vi "Get ObjFlags.vi"(11 "Object Type in":refnum<class "Object Type Base.lvclass">) -> (1 "Set?":bool, 2 "ObjFlags":u32, 3 "Object Type out":refnum<class "Object Type Base.lvclass">)   [LabVIEW 2024, in "EDS.lvlib" / "Object Type Base.lvclass"]
uses:
  Object Type Base.lvclass
  Object Type Base.lvclass/Object Type Base.ctl
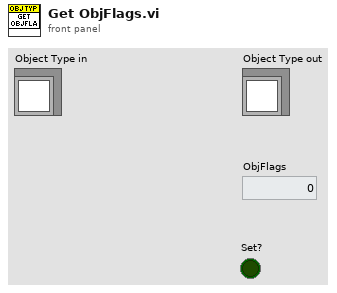
[diagram p1: front panel]
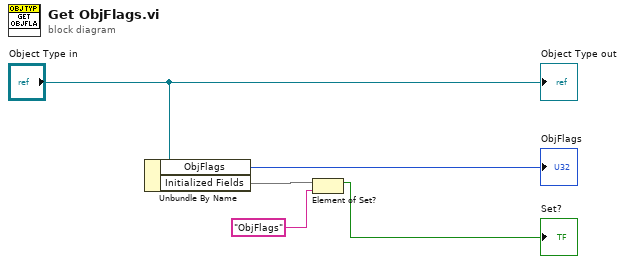
[diagram p0: block diagram]
diagram:
  n1 = Unbundle By Name("Object Type in") -> ("ObjFlags"=→"ObjFlags":u32, "Initialized Fields"=w3:set{string})
  n2 = Element of Set?(10:"ObjFlags" ("element"), 11:w3) -> (3:→"Set?":bool)
  "Object Type out" <- "Object Type in"
